vi "GuiUpdate.vi"(7 "GuiRef":T2={"StringOut"=refnum, "AbortOnFail"=refnum, "SN"=refnum, "SN_Length"=refnum, "TestResult"=refnum, "CycleTime"=refnum, "ErrorCode"=refnum, "UUTStatus"=refnum, "DataBaseEnable?"=refnum, "DUTModel"=refnum, "FixtureID"=refnum, "OperatorID"=refnum, "SNReady"=refnum, "StopSlot"=refnum, "NextStep"=refnum, "PassYeild"=refnum, "Failed"=refnum, "Passed"=refnum, "Tested"=refnum, "TestItemsCtl"={"StepName"="", "TestEnable"=FALSE, "LoopCount"=0, "StopOnFail"=FALSE, "Index"=0, "TestName"="", "通道"="", "参数"="", "TimeStart"=0}, "ProcessBar"=refnum, "Slot"=enum."Slot1", "Row"=3, "States"=refnum, "TestMode"=refnum, "循环次数-DUT"=refnum, "波形图"=refnum, "产品型号"=refnum, "子面板"=refnum, "测试失败项目"=refnum, "测试结果"=refnum, "DUT"=refnum, "Starttime"=refnum, "SlotReady"=refnum, "版本信息"=refnum}, 8 "error in":errorcluster, 9 "States":T1=enum."PostUUT") -> (0 "error out":errorcluster, 2 "PASS/FAIL":bool)   [LabVIEW 2013]
uses:
  SysControl/Reference.ctl
  SysControl/TestItemsCTL.ctl
  SysControl/Slot.ctl
  SysControl/States.ctl
  SysControl/LEDState.ctl
  SysControl/Setup.ctl
  SourceCode/GlobalValue.vi
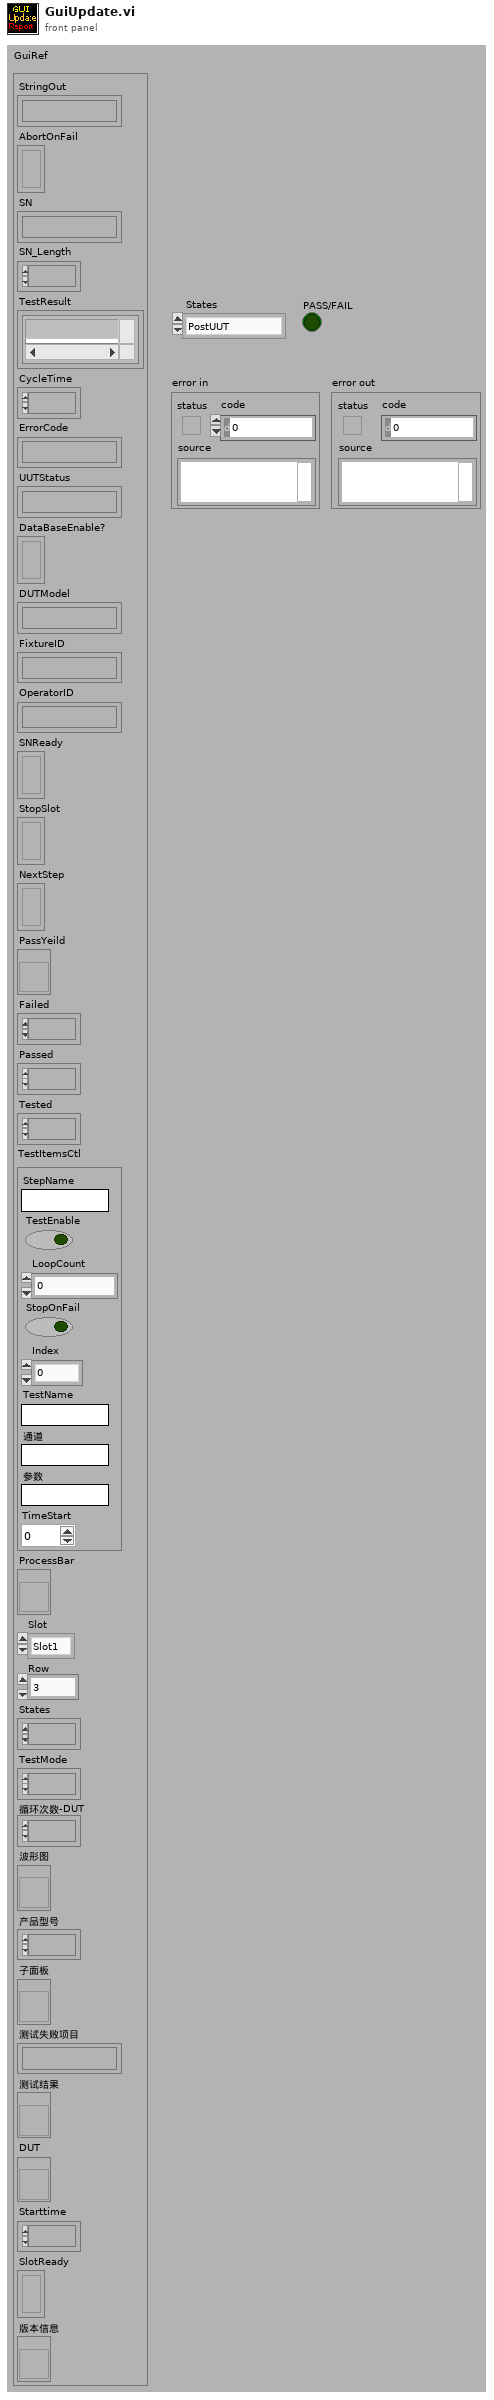
[diagram p1: front panel]
types:
  T1 = typedef "States.ctl" = enum16{"Init", "PreUUT", "Idle", "SetUp", "TestSequence", "PostUUT", "StopTest", "Debug Mode", "Selection Mode", "Loop Mode", "Error", "Wait"}
  T2 = typedef "Reference.ctl" = cluster{"StringOut":refnum<vi>, "AbortOnFail":refnum<vi>, "SN":refnum<vi>, "SN_Length":refnum<vi>, "TestResult":refnum<vi>, "CycleTime":refnum<vi>, "ErrorCode":refnum<vi>, "UUTStatus":refnum<vi>, "DataBaseEnable?":refnum<vi>, "DUTModel":refnum<vi>, "FixtureID":refnum<vi>, "OperatorID":refnum<vi>, "SNReady":refnum<vi>, "StopSlot":refnum<vi>, "NextStep":refnum<vi>, "PassYeild":refnum<vi>, "Failed":refnum<vi>, "Passed":refnum<vi>, "Tested":refnum<vi>, "TestItemsCtl":T3, "ProcessBar":refnum<vi>, "Slot":T4, "Row":u32, "States":refnum<vi>, "TestMode":refnum<vi>, "循环次数-DUT":refnum<vi>, "波形图":refnum<vi>, "产品型号":refnum<vi>, "子面板":refnum<vi>, "测试失败项目":refnum<vi>, "测试结果":refnum<vi>, "DUT":refnum<vi>, "Starttime":refnum<vi>, "SlotReady":refnum<vi>, "版本信息":refnum<vi>}
  T3 = typedef "TestItemsCTL.ctl" = cluster{"StepName":string, "TestEnable":bool, "LoopCount":i32, "StopOnFail":bool, "Index":u32, "TestName":string, "通道":string, "参数":string, "TimeStart":u32}
  T4 = typedef "Slot.ctl" = enum16{"Slot1", "Slot2", "Slot3", "Slot4"}
  T5 = enum8{"Enabled", "Disabled", "Disabled and Grayed Out"}
  T6 = typedef "LEDState.ctl" = enum16{"默认", "闪烁", "停止闪烁", "真", "假"}
  T7 = typedef "Setup.ctl" = cluster{"TestedNum":u32, "PassedNum":u32, "FailedNum":u32, "Slot1TestedNum":u32, "Slot2TestedNum":u32, "Slot3TestedNum":u32, "Slot4TestedNum":u32, "GuiVer":string, "LimitFileVer":string, "Login Name":string, "Password":string, "SN_Head":string, "SN_Length":i32, "AbortOnFail":bool, "DataBaseEnable?":bool, "FixtureID":string, "ShowSkipStep?":bool}
  T8 = typedef "TestMode.ctl" = enum16{"Production Mode", "Selection Mode", "Debug Mode", "Loop Mode", "Stop Test"}
  T9 = enum16{"Production Mode", "Selection Mode", "Debug Mode", "Loop Mode", "Stop Test"}
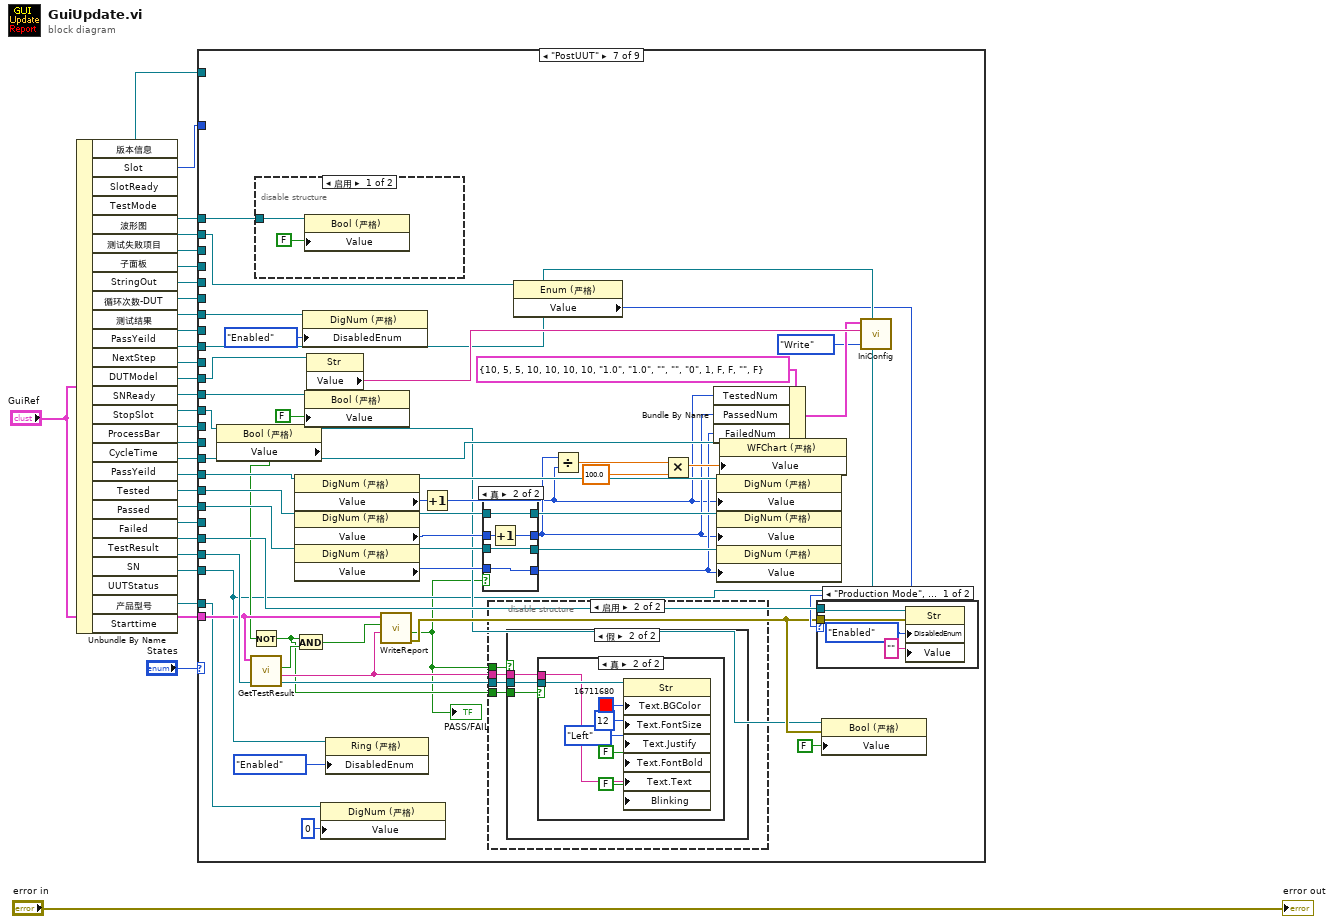
[diagram p0: block diagram]
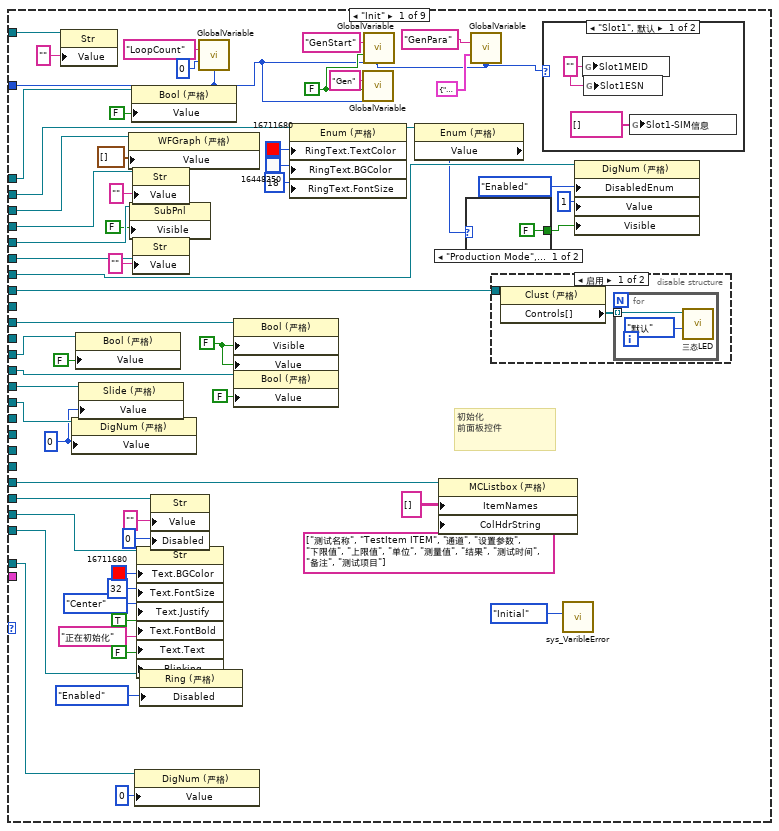
[diagram p2: hidden frame]
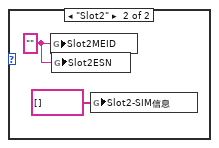
[diagram p3: hidden frame]
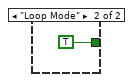
[diagram p4: hidden frame]
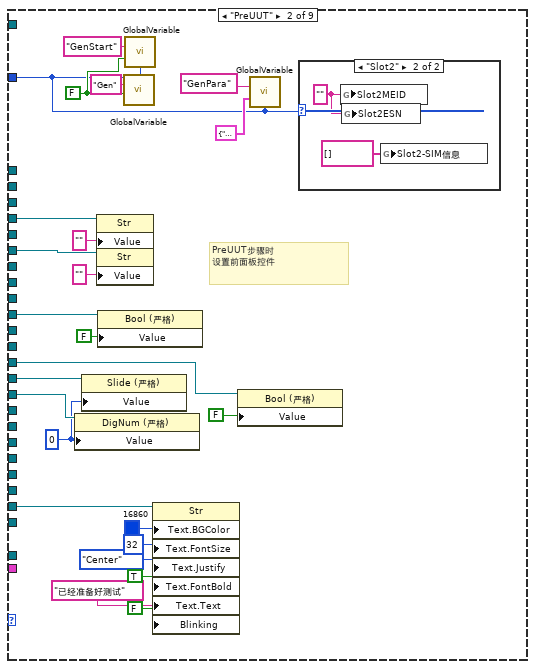
[diagram p6: hidden frame]
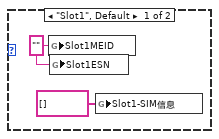
[diagram p7: hidden frame]
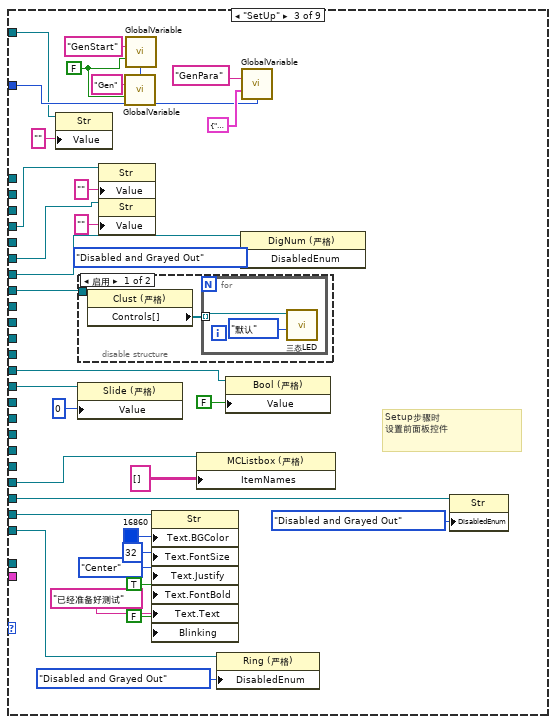
[diagram p8: hidden frame]
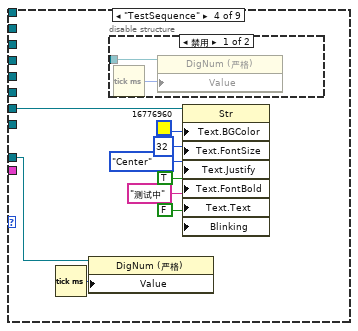
[diagram p10: hidden frame]
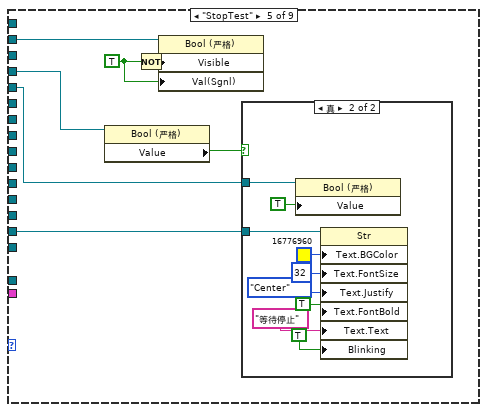
[diagram p12: hidden frame]
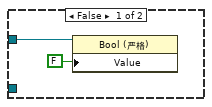
[diagram p13: hidden frame]
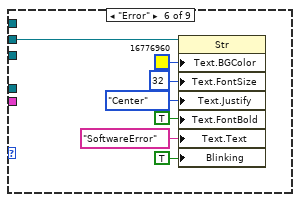
[diagram p14: hidden frame]
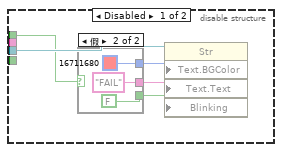
[diagram p17: hidden frame]
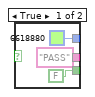
[diagram p18: hidden frame]
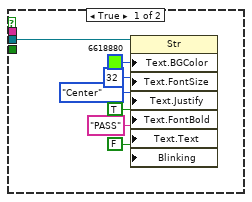
[diagram p19: hidden frame]
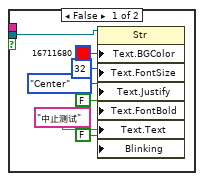
[diagram p20: hidden frame]
diagram:
  n1 = Unbundle By Name("GuiRef") -> ("版本信息"=w1:refnum<vi>, "Slot"=w2:T4, "SlotReady"=w3:refnum<vi>, "TestMode"=w5:refnum<vi>, "波形图"=w6:refnum<vi>, "测试失败项目"=w7:refnum<vi>, "子面板"=w8:refnum<vi>, "StringOut"=w9:refnum<vi>, "循环次数-DUT"=w12:refnum<vi>, "测试结果"=w13:refnum<vi>, "PassYeild"=w15:refnum<vi>, "NextStep"=w16:refnum<vi>, "DUTModel"=w18:refnum<vi>, "SNReady"=w21:refnum<vi>, "StopSlot"=w11:refnum<vi>, "ProcessBar"=w20:refnum<vi>, "CycleTime"=w19:refnum<vi>, "PassYeild"=w25:refnum<vi>, "Tested"=w24:refnum<vi>, "Passed"=w23:refnum<vi>, "Failed"=w22:refnum<vi>, "TestResult"=w27:refnum<vi>, "SN"=w29:refnum<vi>, "UUTStatus"=w28:refnum<vi>, "产品型号"=w10:refnum<vi>, "Starttime"=w4:refnum<vi>)
  n2 = case shown="\"PostUUT\"" "States" {
    tunnel: w29 -> [w85 _ w152 _ _ _ w218 _ _]
    tunnel: w28 -> [w58 w109 w138 w164 w179 w191 w245 _ w325]
    tunnel: w27 -> [w78 _ w155 _ _ _ _ _ _]
    tunnel: w25 -> [_ _ _ _ _ _ w231 _ w306]
    tunnel: w24 -> [_ _ _ _ _ _ w243 _ w322]
    tunnel: w23 -> [_ _ _ _ _ _ w242 _ w321]
    tunnel: w22 -> [_ _ _ _ _ _ w244 _ w323]
    tunnel: w20 -> [w84 w120 w157 _ _ _ _ _ _]
    tunnel: w19 -> [w83 w119 _ _ _ _ _ _ _]
    tunnel: w21 -> [w81 _ _ _ w174 _ w229 _ w304]
    tunnel: w18 -> [_ _ _ _ _ _ w228 _ _]
    tunnel: "GuiRef" -> [_ _ _ _ _ _ w220 _ w303]
    tunnel: w16 -> [w80 w106 _ _ w177 _ _ _ _]
    tunnel: w15 -> [_ _ _ _ _ _ w219 _ _]
    tunnel: w13 -> [w67 _ w150 _ _ _ _ _ _]
    tunnel: w12 -> [w75 _ w154 _ _ _ w217 _ _]
    tunnel: w11 -> [w74 w104 w134 _ w175 _ w215 _ _]
    tunnel: w10 -> [w72 _ w149 _ _ _ w199 _ _]
    tunnel: w9 -> [w70 w116 w147 _ _ _ _ _ _]
    tunnel: w8 -> [w69 _ _ _ _ _ _ _ _]
    tunnel: w7 -> [w65 w114 w145 _ _ _ _ _ _]
    tunnel: w6 -> [w56 _ _ _ _ _ _ _ _]
    tunnel: w5 -> [w51 _ _ _ _ _ w208 _ _]
    tunnel: w4 -> [w48 _ _ w162 _ _ w213 _ _]
    tunnel: w3 -> [w43 _ _ _ _ _ w209 _ w301]
    tunnel: w2 -> [w32 w98 w128 _ _ _ _ _ _]
    tunnel: w1 -> [w31 _ w126 _ _ _ _ _ _]
    frame "Init" {
      w38 = FALSE ("Value")
      w50 = FALSE ("可见")
      w82 = 0 ("Value")
      # "初始化\n前面板控件"
      n3 = property class="Str"(reference=w31, "Value"="" ("值")) -> ()  [unwired: 1 in, 2 out]
      n4 = property class="DigNum (严格)"(reference=w83, "Value"=w82) -> ()  [unwired: 1 in, 2 out]
      n5 = property class="Bool (严格)"(reference=w81, "Value"=FALSE) -> ()  [unwired: 1 in, 2 out]
      n6 = property class="Slide (严格)"(reference=w84, "Value"=w82) -> ()  [unwired: 1 in, 2 out]
      n7 = property class="WFGraph (严格)"(reference=w56, "Value"=waveform(dbl)[] [] ("Fail项波形图2")) -> ()  [unwired: 1 in, 2 out]
      n8 = property class="SubPnl"(reference=w69, "Visible"=FALSE ("可见")) -> ()  [unwired: 1 in, 2 out]
      n9 = property class="Bool (严格)"(reference=w43, "Value"=FALSE) -> ()  [unwired: 1 in, 2 out]
      n10 = property class="Str"(reference=w65, "Value"="" ("值")) -> ()  [unwired: 1 in, 2 out]
      n11 = property class="Str"(reference=w70, "Value"="" ("值")) -> ()  [unwired: 1 in, 2 out]
      n12 = property class="DigNum (严格)"(reference=w48, "Value"=u32 0 ("值")) -> ()  [unwired: 1 in, 2 out]
      n13 = property on="Property Node" class="Str"(reference=w58, "Text.BGColor"=u32 16711680 ("Color Box 2"), "Text.FontSize"=u32 32 ("文本.字体:字号"), "Text.Justify"=enum16{"Left", "Center", "Right"}."Center" ("文本.调整"), "Text.FontBold"=TRUE ("文本.字体:粗体"), "Text.Text"="正在初始化", "Blinking"=FALSE) -> ()  [unwired: 1 in, 2 out]
      n14 = property class="Ring (严格)"(reference=w72, "Disabled"=T5."Enabled" ("禁用")) -> ()  [unwired: 1 in, 2 out]
      n15 = property class="Str"(reference=w85, "Value"="", "Disabled"=u8 0) -> ()  [unwired: 1 in, 2 out]
      n16 = call "GlobalVariable.vi"("Name"="LoopCount", "ValueIn"=0 ("值"), "Slot"=w32) -> ()  [unwired: 9 in, 4 out]
      n17 = property class="Bool (严格)"(reference=w80, "Visible"=w50, "Value"=w50) -> ()  [unwired: 1 in, 2 out]
      n18 = property class="Bool (严格)"(reference=w74, "Value"=FALSE) -> ()  [unwired: 1 in, 2 out]
      n19 = property on="属性节点" class="Enum (严格)"(reference=w51, "RingText.TextColor"=u32 16711680 ("Color Box"), "RingText.BGColor"=u32 16448250 ("Color Box"), "RingText.FontSize"=u32 18 ("下拉列表文本.字体:字号")) -> (reference out=w37:refnum<vi>)  [unwired: 1 in, 1 out]
      n20 = call "GlobalVariable.vi"("Name"="Gen", "ValueIn"=w38, "Slot"=w32) -> ()  [unwired: 9 in, 4 out]
      n21 = call "GlobalVariable.vi"("Name"="GenStart", "ValueIn"=w38, "Slot"=w32) -> ()  [unwired: 9 in, 4 out]
      n22 = property on="属性节点" class="Enum (严格)"(reference=w37) -> ("Value"=w36:T8)  [unwired: 1 in, 2 out]
      n23 = property class="MCListbox (严格)"(reference=w78, "ItemNames"=string[][] [] ("项名"), "ColHdrString"=string[] ["测试名称", "TestItem ITEM", "通道", "设置参数", "下限值", "上限值", "单位", "测量值", "结果", "测试时间", "备注", "测试项目"] ("列首字符串[]")) -> ()  [unwired: 1 in, 2 out]
      n24 = case shown="\"Production Mode\", 默认" w36 {
        tunnel: [FALSE ("可见") TRUE ("可见")] -> w35
        frame "Production Mode", Default {
        }
        frame "Loop Mode" {
        }
      }
      n25 = call "GlobalVariable.vi"("Name"="GenPara", "ValueIn"=cluster{"CH":tag, "Freq":dbl, "AMP":dbl} {"CH"="Dev1/ao1", "Freq"=0.0, "AMP"=0.0} ("Paras 2"), "Slot"=w32) -> ()  [unwired: 9 in, 4 out]
      n26 = disable-structure shown="启用" {
        disable-tunnel: w67 -> [w95 _]
        frame Enabled {
          n27 = property class="Clust (严格)"(reference=w95) -> ("Controls[]"=w94:refnum<vi>[])  [unwired: 1 in, 2 out]
          n28 = for "For循环" {
            tunnel: w94 -> [w96] mode=indexing
            n29 = call "三态LED.vi"("State"=LEDState."默认", "Ctl引用句柄"=w96) -> ()  [unwired: 4 in, 2 out]
          }
        }
        frame Disabled {
        }
      }
      n30 = case shown="\"Slot1\", 默认" w32 {
        frame "Slot1", Default {
          w89 = "" ("Slot2MEID")
          n31 = global write "GlobalValue.vi" "Slot1MEID"(w89) -> ()
          n32 = global write "GlobalValue.vi" "Slot1ESN"(w89) -> ()
          n33 = global write "GlobalValue.vi" "Slot1-SIM信息"(string[] [] ("Slot2-SIM信息")) -> ()
        }
        frame "Slot2" {
          w91 = "" ("Slot2MEID")
          n34 = global write "GlobalValue.vi" "Slot2MEID"(w91) -> ()
          n35 = global write "GlobalValue.vi" "Slot2ESN"(w91) -> ()
          n36 = global write "GlobalValue.vi" "Slot2-SIM信息"(string[] [] ("Slot2-SIM信息")) -> ()
        }
      }
      n37 = call "sys_VaribleError.vi"("Operation"=enum16{"Initial", "Collect"}."Initial") -> ()  [unwired: 10 in, 1 out]
      n38 = property class="DigNum (严格)"(reference=w75, "DisabledEnum"=T5."Enabled" ("禁用"), "Value"=1 ("值"), "Visible"=w35) -> ()  [unwired: 1 in, 2 out]
    }
    frame "PreUUT" {
      w101 = FALSE ("Value")
      w118 = 0 ("Value")
      # "PreUUT步骤时\n设置前面板控件"
      n39 = property class="DigNum (严格)"(reference=w119, "Value"=w118) -> ()  [unwired: 1 in, 2 out]
      n40 = property class="Slide (严格)"(reference=w120, "Value"=w118) -> ()  [unwired: 1 in, 2 out]
      n41 = property class="Str"(reference=w114, "Value"="" ("值")) -> ()  [unwired: 1 in, 2 out]
      n42 = property class="Str"(reference=w116, "Value"="" ("值")) -> ()  [unwired: 1 in, 2 out]
      n43 = property class="Bool (严格)"(reference=w106, "Value"=FALSE) -> ()  [unwired: 1 in, 2 out]
      n44 = call "GlobalVariable.vi"("Name"="Gen", "ValueIn"=w101) -> ()  [unwired: 10 in, 4 out]
      n45 = call "GlobalVariable.vi"("Name"="GenStart", "ValueIn"=w101, "Slot"=w98) -> ()  [unwired: 9 in, 4 out]
      n46 = property on="Property Node" class="Str"(reference=w109, "Text.BGColor"=u32 16860 ("Color Box 2"), "Text.FontSize"=u32 32 ("文本.字体:字号"), "Text.Justify"=enum16{"Left", "Center", "Right"}."Center" ("文本.调整"), "Text.FontBold"=TRUE ("文本.字体:粗体"), "Text.Text"="已经准备好测试", "Blinking"=FALSE) -> ()  [unwired: 1 in, 2 out]
      n47 = property class="Bool (严格)"(reference=w104, "Value"=FALSE) -> ()  [unwired: 1 in, 2 out]
      n48 = call "GlobalVariable.vi"("Name"="GenPara", "ValueIn"=cluster{"CH":tag, "Freq":dbl, "AMP":dbl} {"CH"="Dev1/ao1", "Freq"=0.0, "AMP"=0.0} ("Paras 2"), "Slot"=w98) -> ()  [unwired: 9 in, 4 out]
      n49 = case shown="\"Slot2\"" w98 {
        frame "Slot1", Default {
          w123 = "" ("Slot2MEID")
          n50 = global write "GlobalValue.vi" "Slot1MEID"(w123) -> ()
          n51 = global write "GlobalValue.vi" "Slot1ESN"(w123) -> ()
          n52 = global write "GlobalValue.vi" "Slot1-SIM信息"(string[] [] ("Slot2-SIM信息")) -> ()
        }
        frame "Slot2" {
          w125 = "" ("Slot2MEID")
          n53 = global write "GlobalValue.vi" "Slot2MEID"(w125) -> ()
          n54 = global write "GlobalValue.vi" "Slot2ESN"(w125) -> ()
          n55 = global write "GlobalValue.vi" "Slot2-SIM信息"(string[] [] ("Slot2-SIM信息")) -> ()
        }
      }
    }
    frame "SetUp" {
      w131 = FALSE ("Value")
      # "Setup步骤时\n设置前面板控件"
      n56 = property class="Str"(reference=w126, "Value"="" ("值")) -> ()  [unwired: 1 in, 2 out]
      n57 = property class="Slide (严格)"(reference=w157, "Value"=0) -> ()  [unwired: 1 in, 2 out]
      n58 = disable-structure shown="启用" {
        disable-tunnel: w150 -> [w159 _]
        frame Enabled {
          n59 = property class="Clust (严格)"(reference=w159) -> ("Controls[]"=w158:refnum<vi>[])  [unwired: 1 in, 2 out]
          n60 = for "For循环" {
            tunnel: w158 -> [w160] mode=indexing
            n61 = call "三态LED.vi"("State"=LEDState."默认", "Ctl引用句柄"=w160) -> ()  [unwired: 4 in, 2 out]
          }
        }
        frame Disabled {
        }
      }
      n62 = property class="Str"(reference=w145, "Value"="" ("值")) -> ()  [unwired: 1 in, 2 out]
      n63 = property class="Str"(reference=w147, "Value"="" ("值")) -> ()  [unwired: 1 in, 2 out]
      n64 = call "GlobalVariable.vi"("Name"="Gen", "ValueIn"=w131, "Slot"=w128) -> ()  [unwired: 9 in, 4 out]
      n65 = call "GlobalVariable.vi"("Name"="GenStart", "ValueIn"=w131, "Slot"=w128) -> ()  [unwired: 9 in, 4 out]
      n66 = property on="Property Node" class="Str"(reference=w138, "Text.BGColor"=u32 16860 ("Color Box 2"), "Text.FontSize"=u32 32 ("文本.字体:字号"), "Text.Justify"=enum16{"Left", "Center", "Right"}."Center" ("文本.调整"), "Text.FontBold"=TRUE ("文本.字体:粗体"), "Text.Text"="已经准备好测试", "Blinking"=FALSE) -> ()  [unwired: 1 in, 2 out]
      n67 = property class="MCListbox (严格)"(reference=w155, "ItemNames"=string[][] [] ("项名")) -> ()  [unwired: 1 in, 2 out]
      n68 = property class="Ring (严格)"(reference=w149, "DisabledEnum"=T5."Disabled and Grayed Out" ("禁用")) -> ()  [unwired: 1 in, 2 out]
      n69 = property class="Bool (严格)"(reference=w134, "Value"=FALSE) -> ()  [unwired: 1 in, 2 out]
      n70 = property class="DigNum (严格)"(reference=w154, "DisabledEnum"=T5."Disabled and Grayed Out" ("禁用")) -> ()  [unwired: 1 in, 2 out]
      n71 = call "GlobalVariable.vi"("Name"="GenPara", "ValueIn"=cluster{"CH":tag, "Freq":dbl, "AMP":dbl} {"CH"="Dev1/ao1", "Freq"=0.0, "AMP"=0.0} ("Paras 2"), "Slot"=w128) -> ()  [unwired: 9 in, 4 out]
      n72 = property class="Str"(reference=w152, "DisabledEnum"=T5."Disabled and Grayed Out" ("禁用")) -> ()  [unwired: 1 in, 2 out]
    }
    frame "TestSequence" {
      n73 = Tick Count (ms)() -> (millisecond timer value=w163:u32)
      n74 = property class="DigNum (严格)"(reference=w162, "Value"=w163) -> ()  [unwired: 1 in, 2 out]
      n75 = disable-structure shown="禁用" {
        disable-tunnel: _ -> [w172 _]
        frame Disabled {
          n76 = Tick Count (ms)() -> (millisecond timer value=w171:u32)
          n77 = property on="Property Node" class="DigNum (严格)"(reference=w172, "Value"=w171) -> ()  [unwired: 1 in, 2 out]
        }
        frame Enabled {
        }
      }
      n78 = property on="Property Node" class="Str"(reference=w164, "Text.BGColor"=u32 16776960 ("Color Box 2"), "Text.FontSize"=u32 32 ("文本.字体:字号"), "Text.Justify"=enum16{"Left", "Center", "Right"}."Center" ("文本.调整"), "Text.FontBold"=TRUE ("文本.字体:粗体"), "Text.Text"="测试中", "Blinking"=FALSE) -> ()  [unwired: 1 in, 2 out]
    }
    frame "StopTest" {
      w176 = TRUE
      n79 = property class="Bool (严格)"(reference=w174) -> ("Value"=w173:bool)  [unwired: 1 in, 2 out]
      n80 = Not(x=w176) -> (.not. x?=w178:bool)
      n81 = property on="属性节点" class="Bool (严格)"(reference=w177, "Visible"=w178, "Val(Sgnl)"=w176) -> ()  [unwired: 1 in, 2 out]
      n82 = case shown="真" w173 {
        tunnel: w179 -> [_ w184]
        tunnel: w175 -> [w181 w183]
        frame False {
          n83 = property class="Bool (严格)"(reference=w181, "Value"=FALSE ("值")) -> ()  [unwired: 1 in, 2 out]
        }
        frame True {
          n84 = property class="Bool (严格)"(reference=w183, "Value"=TRUE ("值")) -> ()  [unwired: 1 in, 2 out]
          n85 = property on="Property Node" class="Str"(reference=w184, "Text.BGColor"=u32 16776960 ("Color Box 2"), "Text.FontSize"=u32 32 ("文本.字体:字号"), "Text.Justify"=enum16{"Left", "Center", "Right"}."Center" ("文本.调整"), "Text.FontBold"=TRUE ("文本.字体:粗体"), "Text.Text"="等待停止", "Blinking"=TRUE) -> ()  [unwired: 1 in, 2 out]
        }
      }
    }
    frame "Error" {
      n86 = property on="Property Node" class="Str"(reference=w191, "Text.BGColor"=u32 16776960 ("Color Box 2"), "Text.FontSize"=u32 32 ("文本.字体:字号"), "Text.Justify"=enum16{"Left", "Center", "Right"}."Center" ("文本.调整"), "Text.FontBold"=TRUE ("文本.字体:粗体"), "Text.Text"="SoftwareError", "Blinking"=TRUE) -> ()  [unwired: 1 in, 2 out]
    }
    frame "PostUUT" {
      n87 = property class="Bool (严格)"(reference=w215) -> (reference out=w201:refnum<vi>, "Value"=w206:bool)  [unwired: 1 in, 1 out]
      n88 = Not(x=w206) -> (.not. x?=w203:bool)
      n89 = call "GetTestResult.vi"("GuiRef"=w220) -> ("FailStep"=w214:string, "PASS/FAIL"=w205:bool)  [unwired: 3 in, 6 out]
      n90 = disable-structure shown="启用" {
        disable-tunnel: w209 -> [w250 _]
        frame Enabled {
          n91 = property class="Bool (严格)"(reference=w250, "Value"=FALSE ("值")) -> ()  [unwired: 1 in, 2 out]
        }
        frame Disabled {
        }
      }
      n92 = property on="Property Node" class="DigNum (严格)"(reference=w243) -> (reference out=w240:refnum<vi>, "Value"=w241:u32)  [unwired: 1 in, 1 out]
      n93 = property on="Property Node" class="DigNum (严格)"(reference=w242) -> (reference out=w236:refnum<vi>, "Value"=w239:u32)  [unwired: 1 in, 1 out]
      n94 = property on="Property Node" class="DigNum (严格)"(reference=w244) -> (reference out=w235:refnum<vi>, "Value"=w238:u32)  [unwired: 1 in, 1 out]
      n95 = And(x=w203, y=w205) -> (x .and. y?=w204:bool)
      n96 = property class="DigNum (严格)"(reference=w217, "DisabledEnum"=T5."Enabled" ("禁用")) -> ()  [unwired: 1 in, 2 out]
      n97 = property class="Bool (严格)"(reference=w229, "Value"=FALSE ("值")) -> ()  [unwired: 1 in, 2 out]
      n98 = property class="Str"(reference=w228) -> ("Value"=w227:string)  [unwired: 1 in, 2 out]
      n99 = property class="DigNum (严格)"(reference=w213, "Value"=u32 0 ("值")) -> ()  [unwired: 1 in, 2 out]
      n100 = property class="Ring (严格)"(reference=w199, "DisabledEnum"=T5."Enabled" ("禁用")) -> ()  [unwired: 1 in, 2 out]
      n101 = call "WriteReport.vi"("StepName"=w214, "Pass/Fail"=w204, "GuiRef"=w220) -> ("error out"=w202:errorcluster, "DBresult"=w198:bool)  [unwired: 6 in, 1 out]
      "PASS/FAIL" <- w198
      n102 = Increment(x=w241) -> (x+1=w223:u32)
      n103 = case shown="真" w198 {
        tunnel: w239 -> [w293 w300]
        tunnel: [w293 w299] -> w224
        tunnel: w238 -> [w295 w298]
        tunnel: [w294 w298] -> w225
        tunnel: [w292 w297] -> w237
        tunnel: w236 -> [w292 w297]
        tunnel: w235 -> [w291 w296]
        tunnel: [w291 w296] -> w234
        frame False {
          n104 = Increment(x=w295) -> (x+1=w294:u32)
        }
        frame True {
          n105 = Increment(x=w300) -> (x+1=w299:u32)
        }
      }
      n106 = disable-structure shown="启用" {
        disable-tunnel: w245 -> [w254 w265]
        disable-tunnel: w198 -> [w252 w266]
        disable-tunnel: w214 -> [_ w264]
        disable-tunnel: w203 -> [_ w263]
        frame Disabled {
          n107 = case shown="假" w252 {
            tunnel: [FALSE ("Blinking") FALSE ("Blinking")] -> w256
            tunnel: ["PASS" ("Text.Text") "FAIL" ("Text.Text")] -> w255
            tunnel: [u32 6618880 ("Color Box 2") u32 16711680 ("Color Box 2")] -> w253
            frame True {
            }
            frame False {
            }
          }
          n108 = property on="Property Node" class="Str"(reference=w254, "Text.BGColor"=w253, "Text.Text"=w255, "Blinking"=w256) -> ()  [unwired: 1 in, 2 out]
        }
        frame Enabled {
          n109 = case shown="假" w266 {
            tunnel: w265 -> [w269 w276]
            tunnel: w264 -> [_ w275]
            tunnel: w263 -> [_ w274]
            frame True {
              n110 = property on="Property Node" class="Str"(reference=w269, "Text.BGColor"=u32 6618880 ("Color Box 2"), "Text.FontSize"=u32 32 ("文本.字体:字号"), "Text.Justify"=enum16{"Left", "Center", "Right"}."Center" ("文本.调整"), "Text.FontBold"=TRUE ("文本.字体:粗体"), "Text.Text"="PASS", "Blinking"=FALSE) -> ()  [unwired: 1 in, 2 out]
            }
            frame False {
              n111 = case shown="真" w274 {
                tunnel: w276 -> [w277 w285]
                tunnel: w275 -> [_ w284]
                frame False {
                  n112 = property on="Property Node" class="Str"(reference=w277, "Text.BGColor"=u32 16711680 ("Color Box 2"), "Text.FontSize"=u32 32 ("文本.字体:字号"), "Text.Justify"=enum16{"Left", "Center", "Right"}."Center" ("文本.调整"), "Text.FontBold"=FALSE ("文本.字体:粗体"), "Text.Text"="中止测试" ("f"), "Blinking"=FALSE) -> ()  [unwired: 1 in, 2 out]
                }
                frame True {
                  n113 = property on="Property Node" class="Str"(reference=w285, "Text.BGColor"=u32 16711680 ("Color Box 2"), "Text.FontSize"=u32 12 ("文本.字体:字号"), "Text.Justify"=enum16{"Left", "Center", "Right"}."Left" ("文本.调整"), "Text.FontBold"=FALSE ("文本.字体:粗体"), "Text.Text"=w284, "Blinking"=FALSE) -> ()  [unwired: 1 in, 2 out]
                }
              }
            }
          }
        }
      }
      n114 = property class="Enum (严格)"(reference=w208) -> ("Value"=w207:T9)  [unwired: 1 in, 2 out]
      n115 = Divide(x=w224, y=w223) -> (x/y=w233:dbl)
      n116 = Multiply(x=w233, y=100.0) -> (x*y=w230:dbl)
      n117 = Bundle By Name(cluster=T7 {"TestedNum"=10, "PassedNum"=5, "FailedNum"=5, "Slot1TestedNum"=10, "Slot2TestedNum"=10, "Slot3TestedNum"=10, "Slot4TestedNum"=10, "GuiVer"="1.0", "LimitFileVer"="1.0", "Login Name"="", "Password"="", "SN_Head"="0", "SN_Length"=1, "AbortOnFail"=FALSE, "DataBaseEnable?"=FALSE, "FixtureID"="", "ShowSkipStep?"=FALSE} ("IN 2"), "TestedNum"=w223, "PassedNum"=w224, "FailedNum"=w225) -> (w222:T7)
      n118 = property on="Property Node" class="DigNum (严格)"(reference=w240, "Value"=w223) -> ()  [unwired: 1 in, 2 out]
      n119 = property on="Property Node" class="DigNum (严格)"(reference=w237, "Value"=w224) -> ()  [unwired: 1 in, 2 out]
      n120 = property on="Property Node" class="DigNum (严格)"(reference=w234, "Value"=w225) -> ()  [unwired: 1 in, 2 out]
      n121 = property on="Property Node" class="WFChart (严格)"(reference=w231, "Value"=w230) -> ()  [unwired: 1 in, 2 out]
      n122 = case shown="\"Production Mode\", 默认" w207 {
        tunnel: w218 -> [w249 _]
        tunnel: w202 -> [w248 _]
        frame "Production Mode", Default {
          n123 = property class="Str"(reference=w249, error in=w248, "DisabledEnum"=T5."Enabled" ("禁用"), "Value"="" ("值")) -> ()  [unwired: 2 out]
        }
        frame "Loop Mode" {
        }
      }
      n124 = property class="Bool (严格)"(reference=w201, error in=w202, "Value"=FALSE ("Blinking")) -> ()  [unwired: 2 out]
      n125 = call "IniConfig.vi"("产品型号"=w199, "PassYeild"=w219, "Operate"=enum16{"Write", "Read"}."Write", "ModelName"=w227, "ConfigIn"=w222) -> ()  [unwired: 1 in, 6 out]
    }
    frame "Wait", Default {
    }
    frame "Loop Mode" {
      n126 = property class="Bool (严格)"(reference=w301, "Value"=TRUE) -> ()  [unwired: 1 in, 2 out]
      n127 = property class="Bool (严格)"(reference=w304, "Value"=TRUE) -> ()  [unwired: 1 in, 2 out]
      n128 = property on="Property Node" class="DigNum (严格)"(reference=w322) -> (reference out=w319:refnum<vi>, "Value"=w320:u32)  [unwired: 1 in, 1 out]
      n129 = property on="Property Node" class="DigNum (严格)"(reference=w321) -> (reference out=w313:refnum<vi>, "Value"=w317:u32)  [unwired: 1 in, 1 out]
      n130 = property on="Property Node" class="DigNum (严格)"(reference=w323) -> (reference out=w312:refnum<vi>, "Value"=w316:u32)  [unwired: 1 in, 1 out]
      n131 = Increment(x=w320) -> (x+1=w310:u32)
      n132 = call "GetTestResult.vi"("GuiRef"=w303) -> ("PASS/FAIL"=w318:bool)  [unwired: 2 in, 8 out]
      n133 = case shown="假" w318 {
        tunnel: w317 -> [w331 w338]
        tunnel: [w331 w337] -> w309
        tunnel: w316 -> [w333 w336]
        tunnel: [w332 w336] -> w315
        tunnel: [w330 w335] -> w314
        tunnel: w313 -> [w330 w335]
        tunnel: w312 -> [w329 w334]
        tunnel: [w329 w334] -> w311
        frame False {
          n134 = Increment(x=w333) -> (x+1=w332:u32)
        }
        frame True {
          n135 = Increment(x=w338) -> (x+1=w337:u32)
        }
      }
      n136 = Divide(x=w309, y=w310) -> (x/y=w308:dbl)
      n137 = case shown="真" w318 {
        tunnel: [FALSE ("Blinking") FALSE ("Blinking")] -> w327
        tunnel: ["PASS" ("Text.Text") "FAIL" ("Text.Text")] -> w326
        tunnel: [u32 6618880 ("Color Box 2") u32 16711680 ("Color Box 2")] -> w324
        frame True {
        }
        frame False {
        }
      }
      n138 = Multiply(x=w308, y=1000.0) -> (x*y=w305:dbl)
      n139 = property on="Property Node" class="Str"(reference=w325, "Text.BGColor"=w324, "Text.Text"=w326, "Blinking"=w327) -> ()  [unwired: 1 in, 2 out]
      n140 = property on="Property Node" class="DigNum (严格)"(reference=w319, "Value"=w310) -> ()  [unwired: 1 in, 2 out]
      n141 = property on="Property Node" class="DigNum (严格)"(reference=w314, "Value"=w309) -> ()  [unwired: 1 in, 2 out]
      n142 = property on="Property Node" class="DigNum (严格)"(reference=w311, "Value"=w315) -> ()  [unwired: 1 in, 2 out]
      n143 = property on="Property Node" class="WFChart (严格)"(reference=w306, "Value"=w305) -> ()  [unwired: 1 in, 2 out]
    }
  }
  "error out" <- "error in"
